vi "Basic Then.vi"(8 "error in (no error)":errorcluster) -> (0 "error out":errorcluster)   [LabVIEW 2017, in "Unit Tests.lvlib"]
uses:
  Unit Tests.lvlib
  3b260d09-8f59-4a5c-a4b2-80d4bb780ead.vi
  e06ebc77-16ed-4273-80f2-dc4d26afb9b6.vi
  5d5fb828-b763-44a5-b0e9-5295b35f93e1.vi
  Promise Future/Promise/Promise.lvclass
  E:/Promise/Promise Future/Future/Future.lvclass
  Basic Then Callback.vi
  Promise Future/Future/Write Future.vi
  Promise Future/Promise/Read Future.vi
  Promise Future/Future/Wrapper VI Name.vi
  Promise Future/Future/Then.vi
  Promise Future/Future/Read Value.vi
  Promise Future/Future/Future.lvclass
  <vilib>/addons/_JKI Toolkits/Caraya/classes/Test/Test.lvclass
  <vilib>/addons/_JKI Toolkits/Caraya/classes/Assert/Assert.lvclass
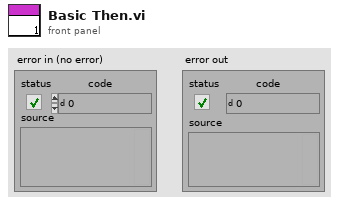
[diagram p1: front panel]
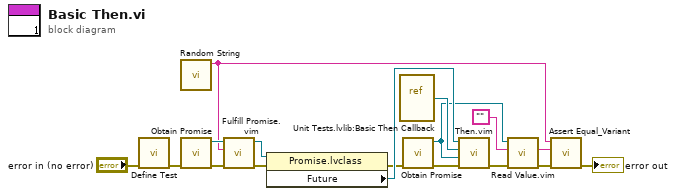
[diagram p0: block diagram]
diagram:
  n1 = call <vilib>:"Define Test.vi"("error in (no error)"="error in (no error)") -> ("error out"=w6:errorcluster)  [unwired: 10 in]
  n2 = call "Random String.vi"() -> ("string"=w1:string)  [unwired: 11 in]
  n3 = call "Obtain Promise.vi"("error in (no error)"=w6) -> ("error out"=w7:errorcluster, "Promise out"=w16:refnum<class "Promise.lvclass">)  [unwired: 8 in, 1 out]
  n4 = call "Fulfill Promise.vim"("error in (no error)"=w7, "Value"=w1, "Promise in"=w16) -> ("error out"=w8:errorcluster, "Promise out"=w4:refnum<class "Promise.lvclass">)  [unwired: 7 in]
  n5 = property class="Promise.lvclass"(reference=w4, error in=w8) -> (error out=w9:errorcluster, "Future"=w15:refnum<class "Future.lvclass">)  [unwired: 1 out]
  n6 = vi-ref "Unit Tests.lvlib:Basic Then Callback.vi"() -> (w17:refnum<vi>)
  n7 = call "Obtain Promise.vi"("error in (no error)"=w9) -> ("error out"=w10:errorcluster, "Promise out"=w3:refnum<class "Promise.lvclass">)  [unwired: 8 in, 1 out]
  n8 = call "Then.vim"("error in (no error)"=w10, "Scope"=w3, "VI"=w17, "Future in"=w15) -> ("error out"=w11:errorcluster)  [unwired: 6 in, 1 out]
  n9 = call "Read Value.vim"("error in (no error)"=w11, "Default Value"="", "Future in"=w3) -> ("error out"=w13:errorcluster, "Value"=w2:string)  [unwired: 5 in, 2 out]
  n10 = call <vilib>:"Assert Equal_Variant.vi"("error in (no error)"=w13, "Y"=w2, "X"=w1) -> ("error out"=→"error out":errorcluster)  [unwired: 8 in]
